vi "Error Query.vi"(6 "Enable Power Meter Error (F:Disable)":bool, 8 "error in (no error)":errorcluster, 11 "VISA resource name":refnum<visa-resource-name>) -> (0 "error out":errorcluster, 1 "Error Description":string, 2 "Error Number":i32[](array[numeric]), 3 "VISA resource name out":refnum<visa-resource-name>)   [LabVIEW 2023, in "Anritsu Signal Analyzer Series.lvlib"]
doc: "Queries the instrument for any errors in the instrument's error queue. It will continue to read errors until all errors have been read from the instrument. Any errors will be returned in the <B>error out</B> control.\n\nThis is an integer in the range of -32768 to +32767. The value zero indicates that there is no error or that no event has occurred.\nA negative number indicates the occurrence of a standard error reserved by SCPI. A positive number indicates the occurrence of an error defined by MS2830A."
uses:
  Anritsu Signal Analyzer Series.lvlib
  <vilib>/Utility/error.llb/Trim Whitespace One-Sided.vi
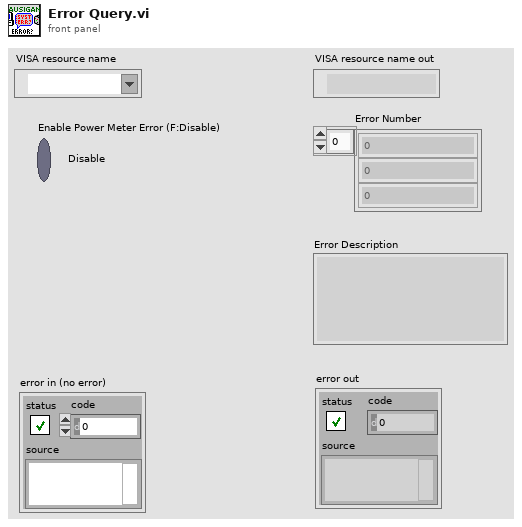
[diagram p1: front panel]
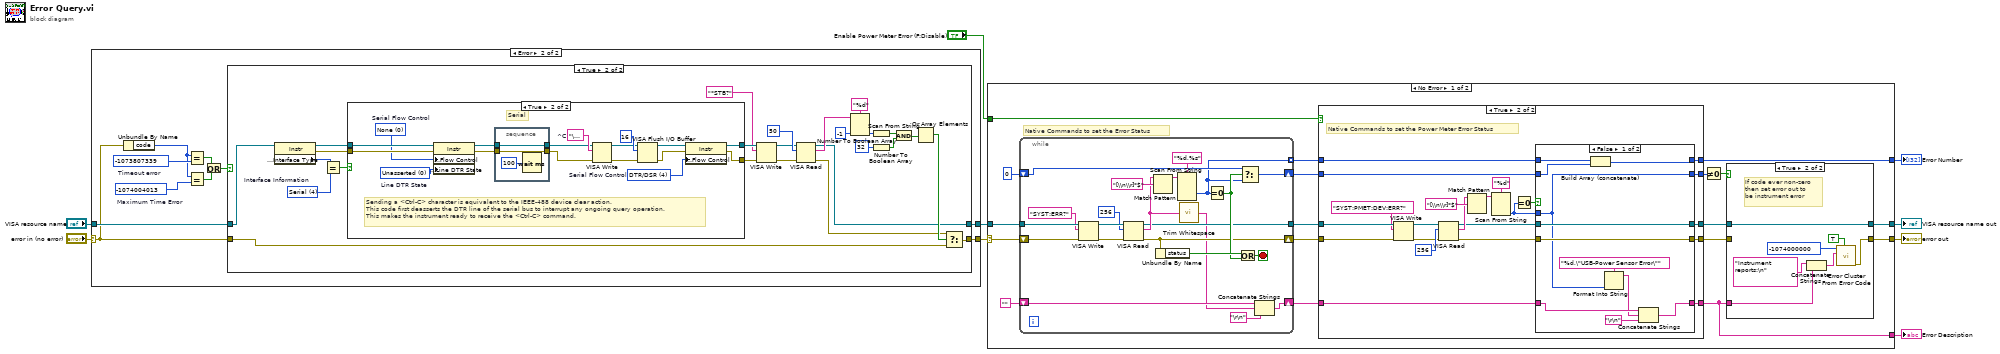
[diagram p0: block diagram]
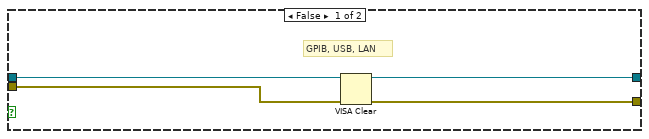
[diagram p4: hidden frame]
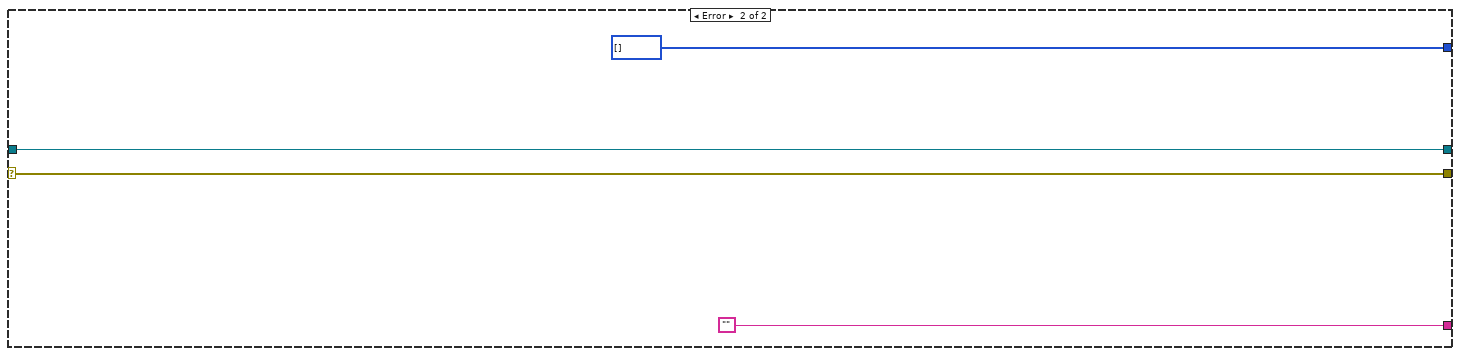
[diagram p8: hidden frame]
diagram:
  n1 = case shown="Error" "error in (no error)" {
    selector: "error in (no error)" -> [w10 w18]
    tunnel: "VISA resource name" -> [w11 w21]
    tunnel: [w11 w19] -> w9
    tunnel: [w10 w17] -> w8
    frame No Error {
    }
    frame Error {
      w15 = -1074004013  # Maximum Time Error
      w20 = -1073807339  # Timeout error
      n2 = Unbundle By Name(w18) -> ("code"=w16:i32)
      n3 = Equal?(x=w16, y=w20) -> (x = y?=w12:bool)
      n4 = Equal?(x=w16, y=w15) -> (x = y?=w14:bool)
      n5 = Or(x=w12, y=w14) -> (x .or. y?=w13:bool)
      n6 = case shown="True" w13 {
        tunnel: w21 -> [w23 w36]
        tunnel: [w23 w26] -> w19
        tunnel: w18 -> [w22 w44]
        tunnel: [w22 w43] -> w17
        frame False {
          # "Error code not a timeout, so best to pass on to user."
        }
        frame True {
          w37 = u16 4 items=["GPIB"=1, "VXI"=2, "GPIB-VXI"=3, "Serial"=4, "PXI"=5, "TCPIP"=6, "USB"=7]  # Interface Information
          n7 = property on="Property Node" class="Instr"(reference=w36) -> (reference out=w41:refnum<visa-resource-name>, error out=w39:errorcluster, "Interface Information:Interface Type"=w38:u16)  [unwired: 1 in]
          n8 = Equal?(x=w38, y=w37) -> (x = y?=w40:bool)
          n9 = case shown="True" w40 {
            tunnel: w39 -> [w49 w68]
            tunnel: [w51 w65] -> w29
            tunnel: [w50 w64] -> w28
            tunnel: w41 -> [w52 w69]
            frame False {
              # "GPIB, USB, LAN"
              n10 = VISA Clear(VISA resource name=w52, error in (no error)=w49) -> (VISA resource name out=w51:refnum<visa-resource-name>, error out=w50:errorcluster)
            }
            frame True {
              w66 = u16 4 items=["None"=0, "XON/XOFF"=1, "RTS/CTS"=2, "DTR/DSR"=4]  # Serial Flow Control
              w59 = u16 0 items=["None"=0, "XON/XOFF"=1, "RTS/CTS"=2, "DTR/DSR"=4]  # Serial Flow Control
              w67 = "\u0003"  # ^C
              w60 = i16 0 items=["Unknown"=-1, "Unasserted"=0, "Asserted"=1]  # Line DTR State
              # "Sending a <Ctrl-C> character is equivalent to the IEEE-488 device clear action.  \nThis code first deasserts the DTR line of the serial bus to interrupt any ongoing query operation.  \nThis makes the instrument ready to receive the <Ctrl-C> command."
              # "Serial"
              n11 = property on="Property Node" class="Instr"(reference=w69, error in=w68, "Serial Settings:Flow Control"=w59, "Serial Settings:Modem Line Settings:Line DTR State"=w60) -> (reference out=w63:refnum<visa-resource-name>, error out=w62:errorcluster)
              n12 = stacked-sequence {
                tunnel: [w71] -> w58
                tunnel: w63 -> [w71]
                tunnel: [w70] -> w57
                tunnel: w62 -> [w70]
                frame #0 {
                  n13 = Wait (ms)(milliseconds to wait=u32 100) -> ()  [unwired: 1 out]
                }
              }
              n14 = VISA Write(VISA resource name=w58, write buffer=w67, error in (no error)=w57) -> (VISA resource name out=w54:refnum<visa-resource-name>, error out=w53:errorcluster)  [unwired: 1 out]
              n15 = VISA Flush I/O Buffer(VISA resource name=w54, mask (16)=u16 16, error in (no error)=w53) -> (VISA resource name out=w56:refnum<visa-resource-name>, error out=w55:errorcluster)
              n16 = property on="Property Node" class="Instr"(reference=w56, error in=w55, "Serial Settings:Flow Control"=w66) -> (reference out=w65:refnum<visa-resource-name>, error out=w64:errorcluster)
            }
          }
          n17 = VISA Write(VISA resource name=w29, write buffer="*STB?" ("_Command"), error in (no error)=w28) -> (VISA resource name out=w30:refnum<visa-resource-name>, error out=w31:errorcluster)  [unwired: 1 out]
          n18 = VISA Read(VISA resource name=w30, byte count=u32 50 ("byte count (0)"), error in (no error)=w31) -> (VISA resource name out=w26:refnum<visa-resource-name>, read buffer=w33:string, error out=w25:errorcluster)  [unwired: 1 out]
          n19 = Scan From String(format string="%d" ("Format String"), input string=w33, default 1=-1 ("_Default")) -> (output 1=w27:i32)  [unwired: 2 in, 3 out]
          n20 = Number To Boolean Array(number=w27) -> (Boolean array=w45:bool[])
          n21 = Number To Boolean Array(number=32) -> (Boolean array=w47:bool[])
          n22 = And(x=w45, y=w47) -> (x .and. y?=w46:bool[])
          n23 = Or Array Elements(Boolean array=w46) -> (logical OR=w42:bool)
          n24 = Select(t=w25, s=w42, f=w44) -> (s? t:f=w43:errorcluster)
        }
      }
    }
  }
  n25 = case shown="No Error" w8 {
    selector: w8 -> [w86 w165]
    tunnel: [w84 w168] -> w4
    tunnel: w9 -> [w85 w168]
    tunnel: [w87 w165] -> w5
    tunnel: [w78 "" ("Empty String Constant")] -> w2
    tunnel: [w74 i32[] []] -> w3
    tunnel: "Enable Power Meter Error (F:Disable)" -> [w73 _]
    frame No Error {
      # "Native Commands to set the Error Status"
      n26 = while {
        tunnel: [w147] -> w83
        tunnel: w85 -> [w148]
        shift-right: [w161] -> w79
        shift-left: "" ("Empty String Constant") -> [w163]
        shift-right: [w159] -> w76
        shift-left: 0 -> [w160]
        shift-right: [w146] -> w82
        shift-left: w86 -> [w149]
        tunnel: [w144] -> w77 mode=indexing
        stop <- w164 stop-if-true
        n27 = VISA Write(VISA resource name=w148, write buffer="SYST:ERR?", error in (no error)=w149) -> (VISA resource name out=w156:refnum<visa-resource-name>, error out=w155:errorcluster)  [unwired: 1 out]
        n28 = VISA Read(VISA resource name=w156, byte count=u32 256 ("byte count (0)"), error in (no error)=w155) -> (VISA resource name out=w147:refnum<visa-resource-name>, read buffer=w150:string, error out=w146:errorcluster)  [unwired: 1 out]
        n29 = Match Pattern(string=w150, regular expression="[\\n\\r]*$") -> (before substring=w152:string)  [unwired: 1 in, 3 out]
        n30 = Unbundle By Name(w146) -> ("status"=w158:bool)
        n31 = Scan From String(format string="%d,%s" ("形式文字列"), input string=w152) -> (output 1=w144:i32)  [unwired: 5 in, 3 out]
        n32 = call <vilib>:"Trim Whitespace.vi"("string"=w150) -> ("trimmed string"=w145:string)  [unwired: 1 in]
        n33 = Equal To 0?(x=w144) -> (x = 0?=w157:bool)
        n34 = Or(x=w158, y=w157) -> (x .or. y?=w164:bool)
        n35 = Select(t=w160, s=w157, f=w144) -> (s? t:f=w159:i32)
        n36 = Concatenate Strings(w163, w145, "\r\n" ("End of Line Constant")) -> (w161:string)
      }
      n37 = case shown="True" w73 {
        tunnel: w83 -> [w93 w114]
        tunnel: w82 -> [w92 w113]
        tunnel: [w93 w104] -> w81
        tunnel: [w92 w103] -> w80
        tunnel: w79 -> [w91 w102]
        tunnel: [w91 w101] -> w78
        tunnel: w77 -> [w95 w100]
        tunnel: w76 -> [w94 w99]
        tunnel: [w94 w98] -> w75
        tunnel: [w95 w97] -> w74
        frame False {
        }
        frame True {
          # "Native Commands to set the Power Meter Error Status"
          n38 = VISA Write(VISA resource name=w114, write buffer="SYST:PMET:DEV:ERR?", error in (no error)=w113) -> (VISA resource name out=w115:refnum<visa-resource-name>, error out=w116:errorcluster)  [unwired: 1 out]
          n39 = VISA Read(VISA resource name=w115, byte count=u32 256 ("byte count (0)"), error in (no error)=w116) -> (VISA resource name out=w106:refnum<visa-resource-name>, read buffer=w109:string, error out=w105:errorcluster)  [unwired: 1 out]
          n40 = Match Pattern(string=w109, regular expression="[\\n\\r]*$") -> (before substring=w111:string)  [unwired: 1 in, 3 out]
          n41 = Scan From String(format string="%d" ("形式文字列"), input string=w111) -> (output 1=w96:i32)  [unwired: 3 in, 3 out]
          n42 = Equal To 0?(x=w96) -> (x = 0?=w107:bool)
          n43 = case shown="False" w107 {
            tunnel: w106 -> [w127 w133]
            tunnel: w105 -> [w128 w132]
            tunnel: [w127 w133] -> w104
            tunnel: [w128 w132] -> w103
            tunnel: w102 -> [w125 w129]
            tunnel: [w124 w129] -> w101
            tunnel: w100 -> [w120 w130]
            tunnel: w99 -> [w119 w131]
            tunnel: [w121 w131] -> w98
            tunnel: [w118 w130] -> w97
            tunnel: w96 -> [w121 _]
            frame False {
              n44 = Build Array (concatenate)(w120, w119) -> (w118:i32[])
              n45 = Format Into String(format string="%d,\"USB-Power Sensor Error\"" ("形式文字列"), w121) -> (resulting string=w122:string)  [unwired: 2 in, 1 out]
              n46 = Concatenate Strings(w125, w122, "\r\n" ("End of Line Constant")) -> (w124:string)
            }
            frame True {
            }
          }
        }
      }
      n47 = Not Equal To 0?(x=w75) -> (x != 0?=w88:bool)
      n48 = case shown="True" w88 {
        tunnel: w78 -> [_ w141]
        tunnel: [w135 w137] -> w87
        tunnel: w80 -> [w135 _]
        tunnel: w81 -> [w134 w136]
        tunnel: [w134 w136] -> w84
        frame False {
        }
        frame True {
          # "If code ever non-zero\nthen set error out to\nbe instrument error"
          n49 = Concatenate Strings("Instrument reports:\n" ("Source"), w141) -> (w138:string)
          n50 = call <vilib>:"Error Cluster From Error Code.vi"("show call chain? (False)"=TRUE, "error message (\"\")"=w138, "error code (0)"=-1074000000 ("Code")) -> ("error out"=w137:errorcluster)  [unwired: 6 in]
        }
      }
    }
    frame Error {
    }
  }
  "error out" <- w5
  "VISA resource name out" <- w4
  "Error Number" <- w3
  "Error Description" <- w2
